vi "fmt_formatSingleCell (Numeric).vi"(5 "format string":string="%.6f", 6 "style index":string="0", 7 "Column":string, 8 "error in":errorcluster, 9 "Value":dbl, 10 "Row":i32, 11 "Format buffer":u8[](array[numeric])=[60, 114, 111, 119, 32, 114, 61, 34, 49, 48, 52, 56, 53, 55, 54, 48, 48, 48, 48, 34, 62, 60, 99, 32, 114, 61, 34, 90, 90, 90, 90, 90, 49, 48, 52, 56, 53, 55, 54, 48, 48, 48, 48, 48, 48, 48, 34, 62, 60, 118, 62, 48, 48, 48, 48, 48, 48, 48, 48, 48, 48, 46, 48, 48, 48, 48, 48, 48, 48, 48, 48, 48, 48, 48, 48, 48, 48, 48, 48, 48, 48, 48, 48, 60, 47, 118, 62, 60, 47, 99, 62, 60, 47, 114, 111, 119, 62]) -> (0 "error out":errorcluster, 1 "Formatted data length":i32, 2 "Buffer size":i32, 3 "Formatted buffer":u8[](array[numeric]))   [LabVIEW 2017, in "NI_ExcelFile.lvlib"]
uses:
  <vilib>/express/express shared/NI_ExcelFile/NI_ExcelFile.lvlib
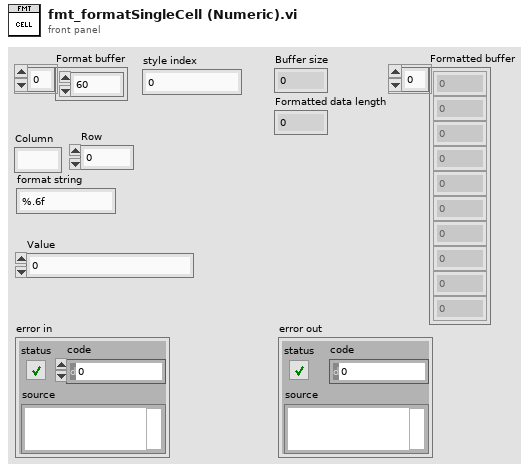
[diagram p1: front panel]
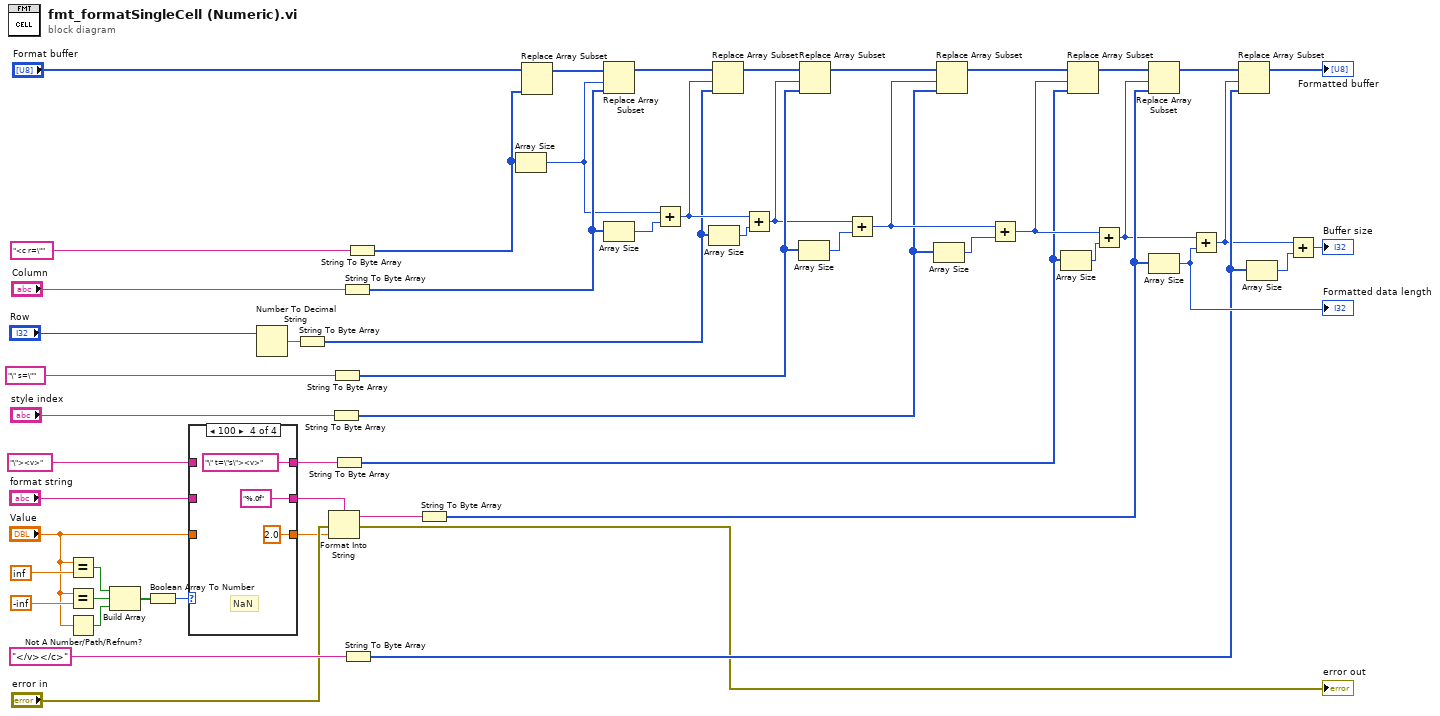
[diagram p0: block diagram]
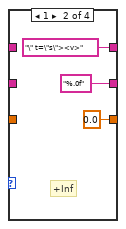
[diagram p3: hidden frame]
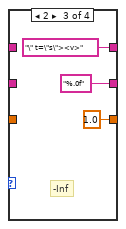
[diagram p4: hidden frame]
diagram:
  n1 = Equal?(x="Value", y=inf) -> (x = y?=w11:bool)
  n2 = Equal?(x="Value", y=-inf) -> (x = y?=w10:bool)
  n3 = Not A Number/Path/Refnum?(number/path/refnum="Value") -> (NaN/Path/Refnum?=w9:bool)
  n4 = Build Array(w11, w10, w9) -> (w8:bool[])
  n5 = Boolean Array To Number(Boolean array=w8) -> (number=w7:u32)
  n6 = case shown="100" w7 {
    tunnel: [w58 "%.0f" ("format string") "%.0f" ("format string") "%.0f" ("format string")] -> w6
    tunnel: "format string" -> [w58 _ _ _]
    tunnel: "Value" -> [w57 _ _ _]
    tunnel: [w57 0.0 ("Value") 1.0 ("Value") 2.0 ("Value")] -> w3
    tunnel: "\"><v>" -> [w56 _ _ _]
    tunnel: [w56 "\" t=\"s\"><v>" "\" t=\"s\"><v>" "\" t=\"s\"><v>"] -> w1
    frame 0, Default {
    }
    frame 1 {
      # "+Inf"
    }
    frame 2 {
      # "-Inf"
    }
    frame 4 {
      # "NaN"
    }
  }
  n7 = Number To Decimal String(number="Row") -> (decimal integer string=w31:string)  [unwired: 1 in]
  n8 = String To Byte Array(string=w31) -> (unsigned byte array=w30:u8[])
  n9 = Format Into String(format string=w6, error in="error in", w3) -> (resulting string=w27:string, error out=→"error out":errorcluster)  [unwired: 1 in]
  n10 = String To Byte Array(string="style index") -> (unsigned byte array=w19:u8[])
  n11 = String To Byte Array(string="\" s=\"") -> (unsigned byte array=w45:u8[])
  n12 = String To Byte Array(string=w1) -> (unsigned byte array=w16:u8[])
  n13 = String To Byte Array(string="Column") -> (unsigned byte array=w52:u8[])
  n14 = String To Byte Array(string="</v></c>") -> (unsigned byte array=w38:u8[])
  n15 = String To Byte Array(string="<c r=\"") -> (unsigned byte array=w49:u8[])
  n16 = String To Byte Array(string=w27) -> (unsigned byte array=w44:u8[])
  n17 = Array Size(array=w49) -> (size(s)=w34:i32)
  n18 = Replace Array Subset(array="Format buffer", new element=w49) -> (w48:u8[])  [unwired: 1 in]
  n19 = Replace Array Subset(array=w48, new element=w52, index=w34) -> (w51:u8[])
  n20 = Array Size(array=w52) -> (size(s)=w43:i32)
  n21 = Add(x=w34, y=w43) -> (x+y=w46:i32)
  n22 = Array Size(array=w30) -> (size(s)=w33:i32)
  n23 = Replace Array Subset(array=w51, new element=w30, index=w46) -> (w47:u8[])
  n24 = Add(x=w46, y=w33) -> (x+y=w42:i32)
  n25 = Array Size(array=w45) -> (size(s)=w41:i32)
  n26 = Replace Array Subset(array=w47, new element=w45, index=w42) -> (w23:u8[])
  n27 = Add(x=w42, y=w41) -> (x+y=w20:i32)
  n28 = Array Size(array=w19) -> (size(s)=w18:i32)
  n29 = Replace Array Subset(array=w23, new element=w19, index=w20) -> (w22:u8[])
  n30 = Add(x=w20, y=w18) -> (x+y=w17:i32)
  n31 = Array Size(array=w16) -> (size(s)=w15:i32)
  n32 = Replace Array Subset(array=w22, new element=w16, index=w17) -> (w21:u8[])
  n33 = Add(x=w17, y=w15) -> (x+y=w14:i32)
  n34 = Replace Array Subset(array=w21, new element=w44, index=w14) -> (w39:u8[])
  n35 = Array Size(array=w44) -> (size(s)=w40:i32)
  "Formatted data length" <- w40
  n36 = Add(x=w14, y=w40) -> (x+y=w36:i32)
  n37 = Replace Array Subset(array=w39, new element=w38, index=w36) -> (→"Formatted buffer":u8[])
  n38 = Array Size(array=w38) -> (size(s)=w37:i32)
  n39 = Add(x=w36, y=w37) -> (x+y=→"Buffer size":i32)
